vi "Status Updated.vi"(8 "error in":errorcluster, 9 "s":bool, 10 "Status":string) -> (0 "error out":errorcluster)   [LabVIEW 2025, in "Full User Interface.lvlib"]
doc: "Send the Status Updated event to any VI registered to listen to events from the owning module.\n_____\nBased on DQMH Project Template 7.0.1.1316."
uses:
  Full User Interface.lvlib
  Status Updated Argument--cluster.ctl
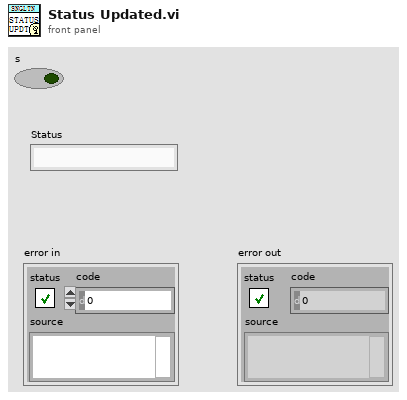
[diagram p1: front panel]
types:
  T1 = typedef "Full User Interface.lvlib/Status Updated Argument--cluster.ctl" = cluster{"Status":string}
  T2 = typedef "Full User Interface.lvlib/Broadcast Events--cluster.ctl" = cluster{"Module Did Init":refnum<user-event>, "Status Updated":refnum<user-event>, "Error Reported":refnum<user-event>, "Module Did Stop":refnum<user-event>, "Update Module Execution Status":refnum<user-event>}
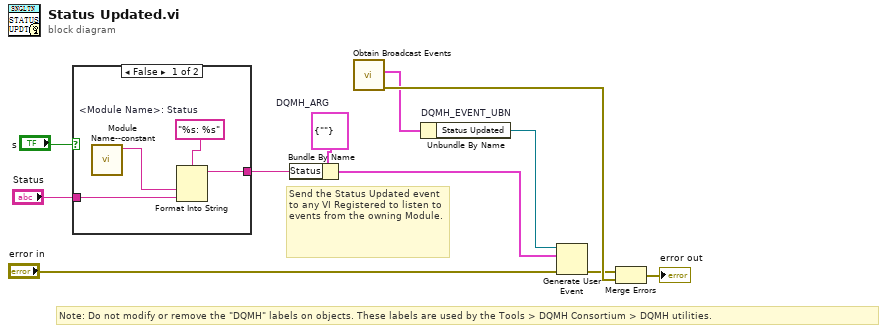
[diagram p0: block diagram]
diagram:
  w5 = T1 {"Status"=""}  # DQMH_ARG
  # "Note: Do not modify or remove the \"DQMH\" labels on objects. These labels are used by the Tools > DQMH Consortium > DQMH utilities."
  # "Send the Status Updated event to any VI Registered to listen to events from the owning Module."
  n1 = case shown="False" "s" {
    tunnel: [w15 w16] -> w3
    tunnel: "Status" -> [w14 w16]
    frame False {
      w12 = "%s: %s"  # <Module Name>: Status
      n2 = call "Module Name--constant.vi"() -> ("Module Name"=w13:string)  [unwired: 11 in]
      n3 = Format Into String(format string=w12, w13, w14) -> (resulting string=w15:string)  [unwired: 2 in, 1 out]
    }
    frame True {
    }
  }
  n4 = Bundle By Name(cluster=w5, "Status"=w3) -> (w4:T1)
  n5 = call "Obtain Broadcast Events.vi"() -> ("error out"=w9:errorcluster, "Full User Interface Broadcast Events"=w7:T2)  [unwired: 10 in]
  n6 = Unbundle By Name "DQMH_EVENT_UBN"(w7) -> ("Status Updated"=w6:refnum<user-event>)
  n7 = Generate User Event(user event=w6, event data cluster=w4, error in="error in") -> (error out=w8:errorcluster)  [unwired: 1 in, 1 out]
  n8 = Merge Errors(w8, w9) -> (→"error out":errorcluster)
